vi "Initialize Control Map.vi"(8 "error in (no error)":errorcluster) -> (0 "error out":errorcluster, 2 "Control Map":map{string, T1[]}(c390))   [LabVIEW 2020, in "MacroAssert.lvlib"]
doc: "Initializes a map of control data."
uses:
  MacroAssert.lvlib
  CTLs/Control Map Control Data.ctl
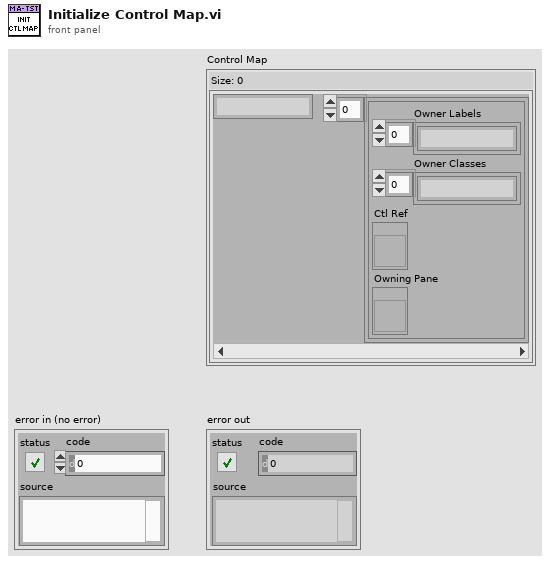
[diagram p1: front panel]
types:
  T1 = typedef "MacroAssert.lvlib/Control Map Control Data.ctl" = cluster{"Owner Labels":string[], "Owner Classes":string[], "Ctl Ref":refnum<vi>, "Owning Pane":refnum<vi>}
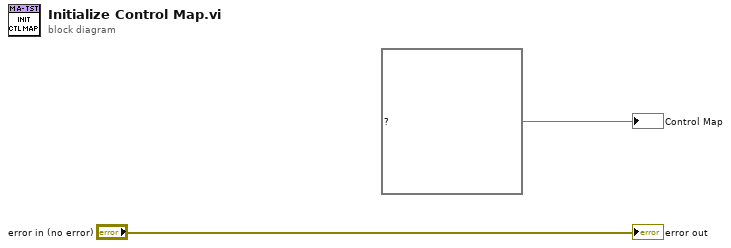
[diagram p0: block diagram]
diagram:
  "error out" <- "error in (no error)"
  "Control Map" <- map{string, T1[]} {} ("map")
